vi "Define Frame.vi"(11 "Matrix":u32[][](array[colorbox])) -> (3 "Array":u8[](array[numeric]))   [LabVIEW 2019, in "LED Matrix Host.lvlib"]
uses:
  LED Matrix Host.lvlib
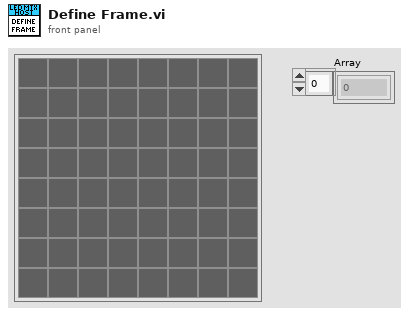
[diagram p1: front panel]
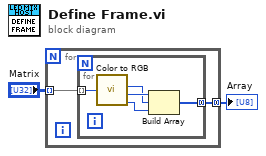
[diagram p0: block diagram]
diagram:
  n1 = for {
    tunnel: "Matrix" -> [w4] mode=indexing
    tunnel: [w3] -> w2 mode=concatenating
    n2 = for {
      tunnel: w4 -> [w9] mode=indexing
      tunnel: [w5] -> w3 mode=concatenating
      n3 = call <vilib>:"Color to RGB.vi"("Color"=w9) -> ("R"=w7:u8, "G"=w8:u8, "B"=w6:u8)  [unwired: 1 out]
      n4 = Build Array(w8, w7, w6) -> (w5:u8[])
    }
  }
  "Array" <- w2
